vi "WaveformServerside.vi"() -> ()   [LabVIEW 2019]
uses:
  <vilib>/measure/NI_MABase.lvlib
panel:
  out "Waveform Graph":waveform(dbl)(graph)
  in  "Stop Wave from Server Side":bool
  out "bytes written":i32
  out "error out":errorcluster
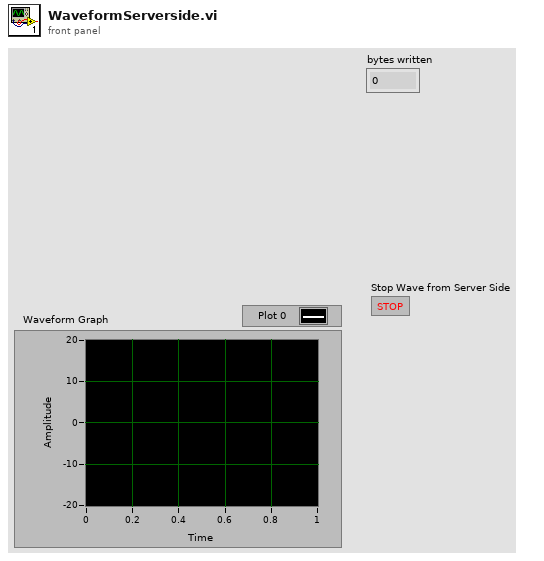
[diagram p1: front panel]
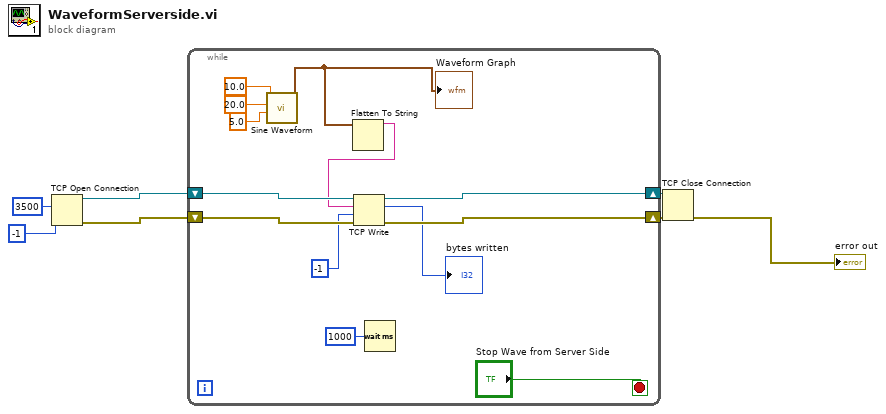
[diagram p0: block diagram]
diagram:
  n1 = TCP Open Connection(remote port or service name=u16 3500, timeout ms (60000)=-1) -> (connection ID=w5:refnum<k5>, error out=w3:errorcluster)  [unwired: 3 in]
  n2 = while {
    shift-right: [w19] -> w4
    shift-left: w5 -> [w20]
    shift-right: [w17] -> w2
    shift-left: w3 -> [w18]
    stop <- "Stop Wave from Server Side" stop-if-true
    n3 = call <vilib>:"Sine Waveform.vi"("phase"=5.0, "amplitude"=20.0, "frequency"=10.0) -> ("signal out"=w8:waveform(dbl))  [unwired: 7 in, 1 out]
    "Waveform Graph" <- w8
    n4 = Flatten To String(anything=w8) -> (data string=w11:string)  [unwired: 3 in, 2 out]
    n5 = TCP Write(connection ID=w20, data in=w11, error in (no error)=w18, 9:-1 ("timeout ms (25000)")) -> (connection ID out=w19:refnum<k5>, bytes written=→"bytes written":i32, error out=w17:errorcluster)
    n6 = Wait (ms)(milliseconds to wait=u32 1000) -> ()  [unwired: 1 out]
  }
  n7 = TCP Close Connection(connection ID=w4, error in (no error)=w2) -> (error out=→"error out":errorcluster)  [unwired: 1 in, 1 out]
